vi "init.vi"(8 "error in (no error)":errorcluster, 10 "Init Data":variant, 11 "Pressure Monitor in":refnum<class "Pressure Monitor.lvclass">) -> (0 "error out":errorcluster, 2 "Channel List":refnum<class "HK Item.lvclass">[](array[class]), 3 "Pressure Monitor out":refnum<class "Pressure Monitor.lvclass">)   [LabVIEW 2024, in "Pressure Monitor.lvclass"]
uses:
  Pressure Monitor.lvclass
  hk-channel-class/hk-channel-class/HK Item/HK Item.lvclass
  Pressure Monitor.lvclass/Pressure Monitor.ctl
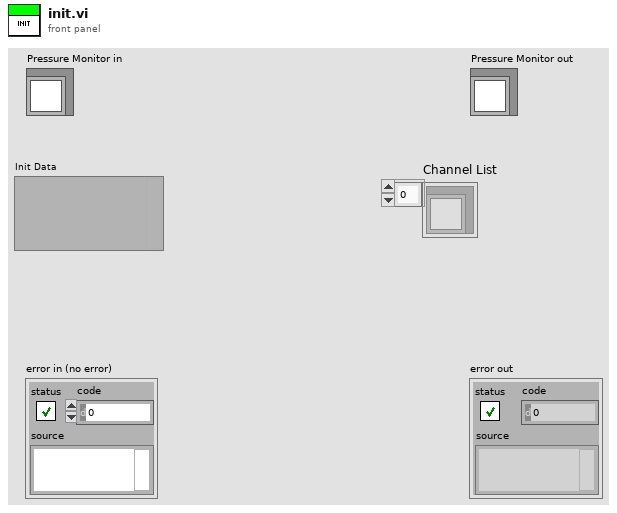
[diagram p1: front panel]
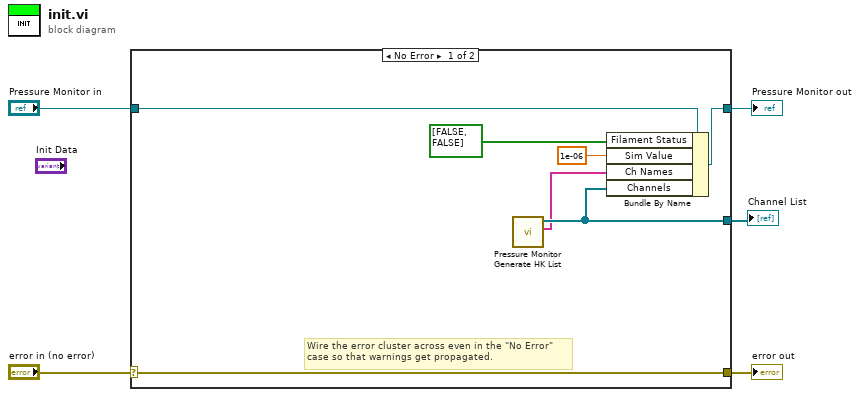
[diagram p0: block diagram]
diagram:
  n1 = case shown="No Error" "error in (no error)" {
    selector: "error in (no error)" -> [w12 w14]
    tunnel: [w12 w14] -> w4
    tunnel: [w10 w13] -> w2
    tunnel: "Pressure Monitor in" -> [w9 w13]
    tunnel: [w11 _] -> w1
    frame No Error {
      # "Wire the error cluster across even in the \"No Error\"\ncase so that warnings get propagated."
      n2 = call "Pressure Monitor Generate HK List.vi"() -> ("Channel Names"=w8:string[], "Channel List"=w11:refnum<class "HK Item.lvclass">[])  [unwired: 10 in]
      n3 = Bundle By Name(cluster=w9, "Filament Status"=bool[] [FALSE, FALSE], "Sim Value"=1e-06, "Ch Names"=w8, "Channels"=w11) -> (w10:refnum<class "Pressure Monitor.lvclass">)
    }
    frame Error {
    }
  }
  "error out" <- w4
  "Pressure Monitor out" <- w2
  "Channel List" <- w1
